vi "Integrate Complex.vi"(3 "integration method":T1 items=["Trapezoidal Rule", "Simpson's Rule", "Simpson's 3/8 Rule", "Bode Rule"], 4 "dx":dbl=1.0 step=0.001 format="%0.4f", 5 "a+bi":cdb[](array[numeric]) format="%0.2f") -> (0 "int(x) img":dbl format="%0.4f", 1 "int(x) real":dbl format="%0.4f", 2 "int(x) cmplx":cdb)   [LabVIEW 2012]
uses:
  <vilib>/Analysis/2dsp.llb/Integral Method.ctl
  <vilib>/Analysis/8numeric.llb/1D Numeric Integration.vi
  <vilib>/Analysis/NI_AALPro.lvlib
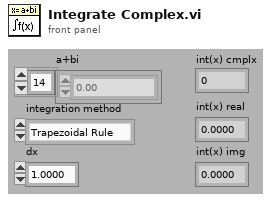
[diagram p1: front panel]
types:
  T1 = typedef "NI_AALPro.lvlib/Integral Method.ctl" = i32
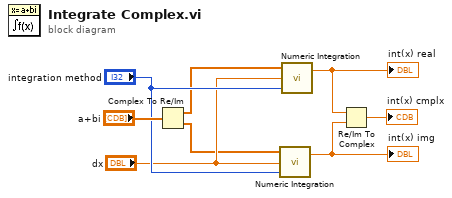
[diagram p0: block diagram]
diagram:
  n1 = Complex To Re/Im(x + iy="a+bi") -> (x=w6:dbl[], y=w4:dbl[])
  n2 = call-poly <vilib>:"Numeric Integration.vi"("integration method"="integration method", "dt"="dx", "Input Array"=w4) -> ("result"=w1:dbl)  [unwired: 1 out]
  "int(x) img" <- w1
  n3 = call-poly <vilib>:"Numeric Integration.vi"("integration method"="integration method", "dt"="dx", "Input Array"=w6) -> ("result"=w3:dbl)  [unwired: 1 out]
  "int(x) real" <- w3
  n4 = Re/Im To Complex(1:w1, 2:w3) -> (0:→"int(x) cmplx":cdb)
